vi "Request Data.vi"(6 "Qualifier":string, 8 "error in":errorcluster, 9 "notifier":refnum<notifier>, 10 "Data to Send":string, 11 "PowerSupply in":refnum<class "PowerSupply.lvclass">) -> (0 "error out":errorcluster, 3 "PowerSupply out":refnum<class "PowerSupply.lvclass">)   [LabVIEW 2019, in "PowerSupply.lvlib" / "PowerSupply.lvclass"]
uses:
  Library/PowerSupply.lvclass
  C:/Users/Public/Documents/Development/builds/Instruments/Instruments.lvlibp/Library/Instruments.lvclass
  C:/Users/Public/Documents/Development/builds/Engine/Monitored Actor.lvlibp/Monitored Actor/Monitored Actor/Monitored Actor.lvclass
  Library/PowerSupply.lvclass/PowerSupply.ctl
  builds/Instruments/Instruments.lvlibp/Accessors/Read Measured.vi
  <vilib>/Utility/error.llb/Error Cluster From Error Code.vi
  builds/Engine/Monitored Actor.lvlibp/Monitored Actor/Monitored Actor/Read Actor Label.vi
  <vilib>/ErrorRing/Error Ring.xnode
  builds/Engine/Engine.lvlibp/Project/Engine.lvclass
  builds/Instruments/Instruments.lvlibp/Library/Instruments.lvclass
  builds/Instruments/Instruments.lvlibp/Private/Polymorphic/Special/Event from String.vi
  builds/Instruments/Instruments.lvlibp
  C:/Users/Public/Documents/Development/builds/Tools/Config.lvlibp/Config.lvclass
  C:/Users/Public/Documents/Development/builds/Engine/Engine.lvlibp/Project/Engine.lvclass
  C:/Users/Public/Documents/Development/builds/Engine/Panel Manager.lvlibp/Panel Actor/Panel Actor.lvclass
  C:/Users/Public/Documents/Development/builds/Engine/Actor Framework.lvlibp/1abvi3w/vi.lib/ActorFramework/Actor/Actor.lvclass
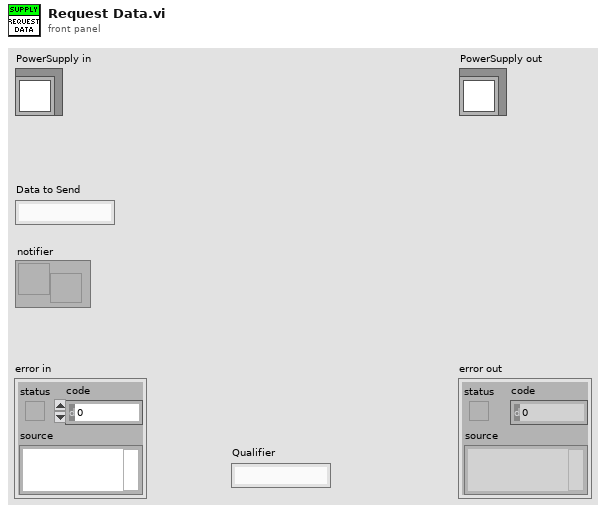
[diagram p1: front panel]
types:
  T1 = typedef "PowerSupply.lvlib/PowerSupply.lvclass/OCP Mode.ctl" = enum16{"Shutdown", "Foldback"}
  T2 = typedef "PowerSupply.lvlib/PowerSupply.lvclass/Sense Point.ctl" = enum16{"Local", "Remote"}
  T3 = cluster{"Timestamp":timestamp, "Description":string, "Data":string}
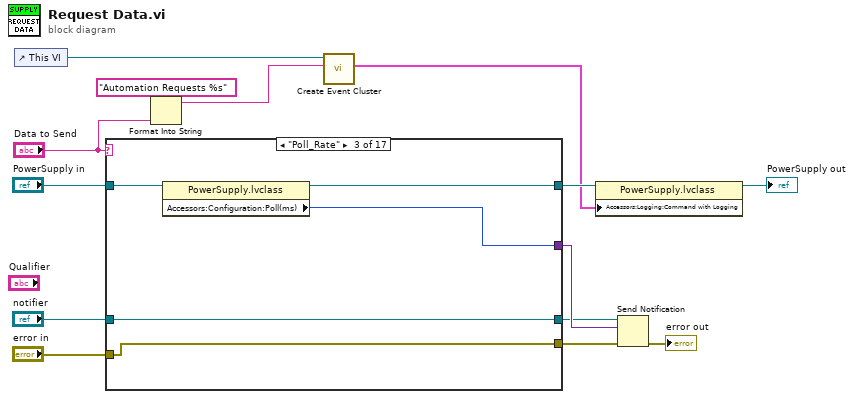
[diagram p0: block diagram]
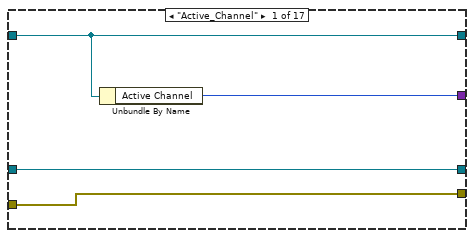
[diagram p2: hidden frame]
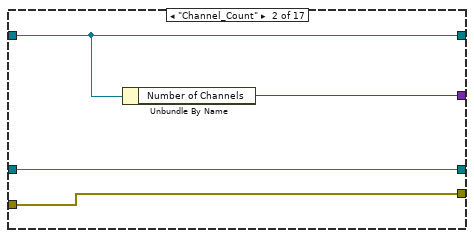
[diagram p3: hidden frame]
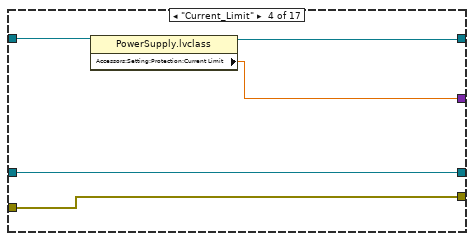
[diagram p4: hidden frame]
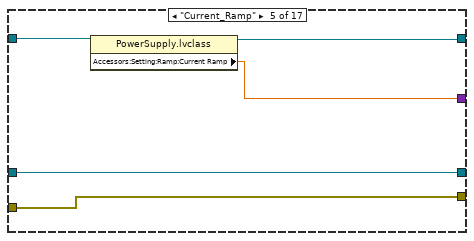
[diagram p5: hidden frame]
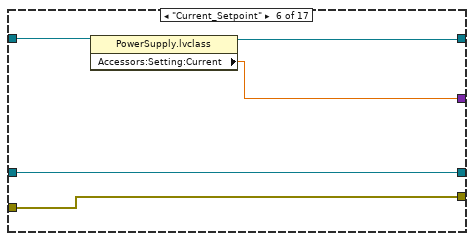
[diagram p6: hidden frame]
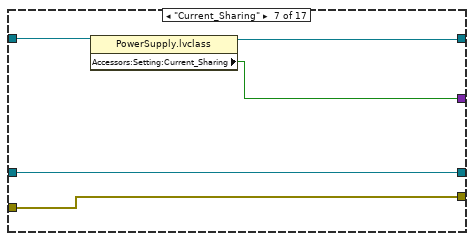
[diagram p7: hidden frame]
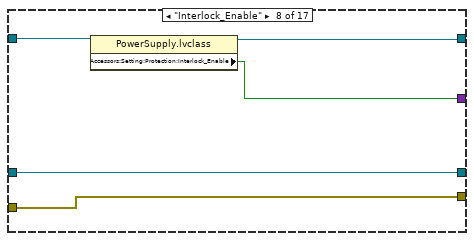
[diagram p8: hidden frame]
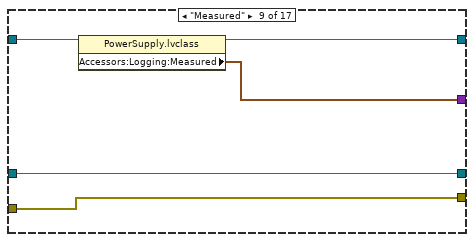
[diagram p9: hidden frame]
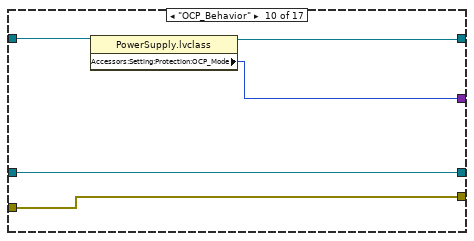
[diagram p10: hidden frame]
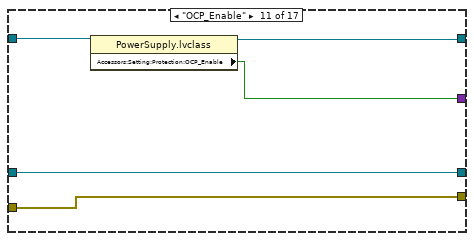
[diagram p11: hidden frame]
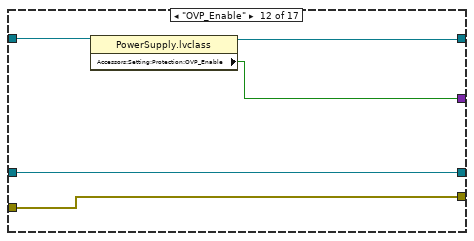
[diagram p12: hidden frame]
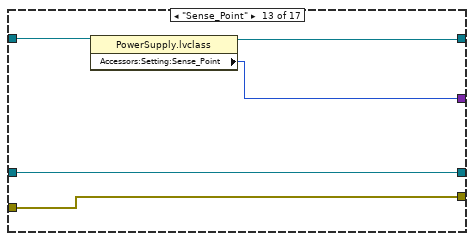
[diagram p13: hidden frame]
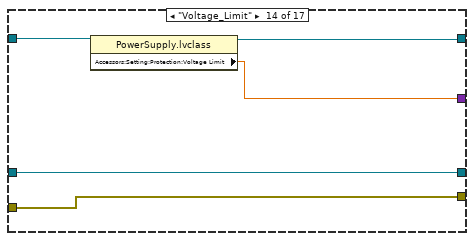
[diagram p14: hidden frame]
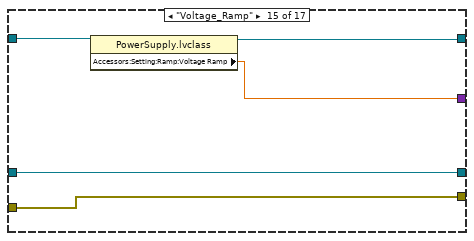
[diagram p15: hidden frame]
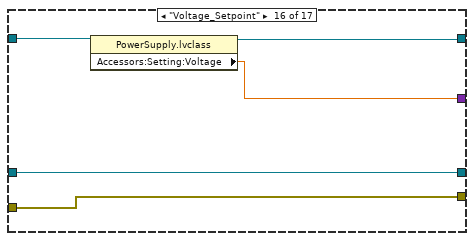
[diagram p16: hidden frame]
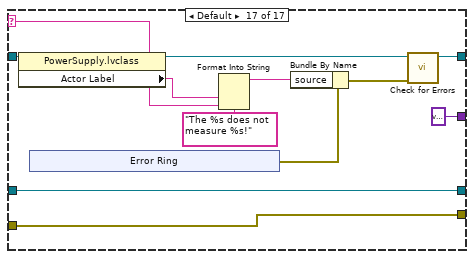
[diagram p17: hidden frame]
diagram:
  n1 = control-ref of="This VI"() -> (w5:refnum<vi>)
  n2 = case shown="\"Poll_Rate\"" "Data to Send" {
    selector: "Data to Send" -> [_ _ _ _ _ _ _ _ _ _ _ _ _ _ _ _ w97]
    tunnel: "PowerSupply in" -> [w18 w22 w25 w32 w37 w42 w47 w52 w57 w62 w67 w72 w77 w82 w87 w92 w96]
    tunnel: [w18 w22 w24 w31 w36 w41 w46 w51 w56 w61 w66 w71 w76 w81 w86 w91 w101] -> w3
    tunnel: [w17 w21 w23 w30 w35 w40 w45 w50 w55 w60 w65 w70 w75 w80 w85 w90 variant] -> w12
    tunnel: "notifier" -> [w16 w20 w27 w29 w34 w39 w44 w49 w54 w59 w64 w69 w74 w79 w84 w89 w103]
    tunnel: [w16 w20 w27 w29 w34 w39 w44 w49 w54 w59 w64 w69 w74 w79 w84 w89 w103] -> w10
    tunnel: "error in" -> [w15 w19 w26 w28 w33 w38 w43 w48 w53 w58 w63 w68 w73 w78 w83 w88 w102]
    tunnel: [w15 w19 w26 w28 w33 w38 w43 w48 w53 w58 w63 w68 w73 w78 w83 w88 w102] -> w8
    frame "Active_Channel" {
      n3 = Unbundle By Name(w18) -> ("Active Channel"=w17:u32)
    }
    frame "Channel_Count" {
      n4 = Unbundle By Name(w22) -> ("Number of Channels"=w21:i32)
    }
    frame "Poll_Rate" {
      n5 = property class="PowerSupply.lvclass"(reference=w25) -> (reference out=w24:refnum<class "PowerSupply.lvclass">, "Accessors:Configuration:Poll(ms)"=w23:u32)  [unwired: 1 in, 1 out]
    }
    frame "Current_Limit" {
      n6 = property class="PowerSupply.lvclass"(reference=w32) -> (reference out=w31:refnum<class "PowerSupply.lvclass">, "Accessors:Setting:Protection:Current Limit"=w30:dbl)  [unwired: 1 in, 1 out]
    }
    frame "Current_Ramp" {
      n7 = property class="PowerSupply.lvclass"(reference=w37) -> (reference out=w36:refnum<class "PowerSupply.lvclass">, "Accessors:Setting:Ramp:Current Ramp"=w35:dbl)  [unwired: 1 in, 1 out]
    }
    frame "Current_Setpoint" {
      n8 = property class="PowerSupply.lvclass"(reference=w42) -> (reference out=w41:refnum<class "PowerSupply.lvclass">, "Accessors:Setting:Current"=w40:dbl)  [unwired: 1 in, 1 out]
    }
    frame "Current_Sharing" {
      n9 = property class="PowerSupply.lvclass"(reference=w47) -> (reference out=w46:refnum<class "PowerSupply.lvclass">, "Accessors:Setting:Current_Sharing"=w45:bool)  [unwired: 1 in, 1 out]
    }
    frame "Interlock_Enable" {
      n10 = property class="PowerSupply.lvclass"(reference=w52) -> (reference out=w51:refnum<class "PowerSupply.lvclass">, "Accessors:Setting:Protection:Interlock_Enable"=w50:bool)  [unwired: 1 in, 1 out]
    }
    frame "Measured" {
      n11 = property class="PowerSupply.lvclass"(reference=w57) -> (reference out=w56:refnum<class "PowerSupply.lvclass">, "Accessors:Logging:Measured"=w55:waveform(dbl)[])  [unwired: 1 in, 1 out]
    }
    frame "OCP_Behavior" {
      n12 = property class="PowerSupply.lvclass"(reference=w62) -> (reference out=w61:refnum<class "PowerSupply.lvclass">, "Accessors:Setting:Protection:OCP_Mode"=w60:T1)  [unwired: 1 in, 1 out]
    }
    frame "OCP_Enable" {
      n13 = property class="PowerSupply.lvclass"(reference=w67) -> (reference out=w66:refnum<class "PowerSupply.lvclass">, "Accessors:Setting:Protection:OCP_Enable"=w65:bool)  [unwired: 1 in, 1 out]
    }
    frame "OVP_Enable" {
      n14 = property class="PowerSupply.lvclass"(reference=w72) -> (reference out=w71:refnum<class "PowerSupply.lvclass">, "Accessors:Setting:Protection:OVP_Enable"=w70:bool)  [unwired: 1 in, 1 out]
    }
    frame "Sense_Point" {
      n15 = property class="PowerSupply.lvclass"(reference=w77) -> (reference out=w76:refnum<class "PowerSupply.lvclass">, "Accessors:Setting:Sense_Point"=w75:T2)  [unwired: 1 in, 1 out]
    }
    frame "Voltage_Limit" {
      n16 = property class="PowerSupply.lvclass"(reference=w82) -> (reference out=w81:refnum<class "PowerSupply.lvclass">, "Accessors:Setting:Protection:Voltage Limit"=w80:dbl)  [unwired: 1 in, 1 out]
    }
    frame "Voltage_Ramp" {
      n17 = property class="PowerSupply.lvclass"(reference=w87) -> (reference out=w86:refnum<class "PowerSupply.lvclass">, "Accessors:Setting:Ramp:Voltage Ramp"=w85:dbl)  [unwired: 1 in, 1 out]
    }
    frame "Voltage_Setpoint" {
      n18 = property class="PowerSupply.lvclass"(reference=w92) -> (reference out=w91:refnum<class "PowerSupply.lvclass">, "Accessors:Setting:Voltage"=w90:dbl)  [unwired: 1 in, 1 out]
    }
    frame Default {
      n19 = property class="PowerSupply.lvclass"(reference=w96) -> (reference out=w95:refnum<class "PowerSupply.lvclass">, "Actor Label"=w94:string)  [unwired: 1 in, 1 out]
      n20 = xnode "Error Ring"() -> ("error out"=w100:errorcluster)
      n21 = Format Into String(format string="The %s does not measure %s!", w94, w97) -> (resulting string=w98:string)  [unwired: 2 in, 1 out]
      n22 = Bundle By Name(cluster=w100, "source"=w98) -> (w99:errorcluster)
      n23 = call "Check for Errors.vi"("error in"=w99, "Engine in"=w95) -> ("Engine out"=w101:refnum<class "PowerSupply.lvclass">)  [unwired: 8 in, 1 out]
    }
  }
  n24 = Format Into String(format string="Automation Requests %s", "Data to Send") -> (resulting string=w4:string)  [unwired: 2 in, 1 out]
  n25 = call-poly "Create Event Cluster.vi"("Value"=w4, "VI Refnum"=w5) -> ("Event Data"=w1:T3)  [unwired: 9 in]
  n26 = property class="PowerSupply.lvclass"(reference=w3, "Accessors:Logging:Command with Logging"=w1) -> (reference out=→"PowerSupply out":refnum<class "PowerSupply.lvclass">)  [unwired: 1 in, 1 out]
  n27 = Send Notification(notification=w12, notifier=w10, error in (no error)=w8) -> (error out=→"error out":errorcluster)  [unwired: 1 out]
